vi "recouple_modes.vi"(10 "Decoupled":sgl[](array[numeric]) format="%#_3f") -> (2 "Output":sgl[](array[numeric]) format="%#_3g")   [LabVIEW 2013]
panel:
  # "Inverse of decouple_modes.vi"
  # "----------XY----------"
  # "----------RxRy----------"
  # "Z"
  # "Rz"
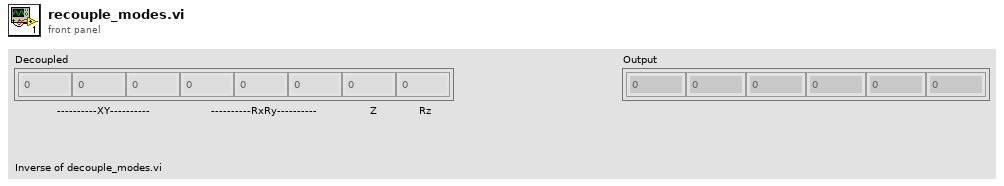
[diagram p1: front panel]
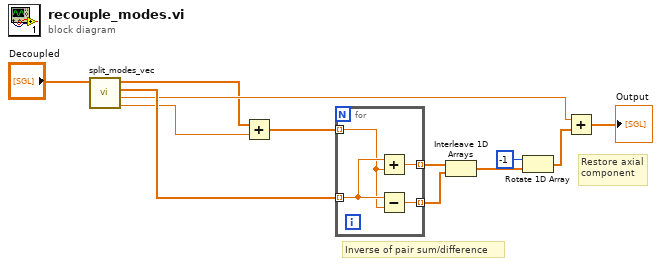
[diagram p0: block diagram]
diagram:
  # "Restore axial\ncomponent"
  # "Inverse of pair sum/difference"
  n1 = call "split_modes_vec.vi"("Decoupled"="Decoupled") -> ("Rz"=w1:sgl, "Z"=w3:sgl, "Rx Ry"=w4:sgl[], "XY"=w2:sgl[])  [unwired: 7 in]
  n2 = Add(x=w2, y=w1) -> (x+y=w7:sgl[])
  n3 = for {
    tunnel: w7 -> [w15] mode=indexing
    tunnel: w4 -> [w16] mode=indexing
    tunnel: [w14] -> w12 mode=indexing
    tunnel: [w13] -> w11 mode=indexing
    n4 = Add(x=w16, y=w15) -> (x+y=w14:sgl)
    n5 = Subtract(x=w16, y=w15) -> (x-y=w13:sgl)
  }
  n6 = Interleave 1D Arrays(w12, w11) -> (w9:sgl[])
  n7 = Rotate 1D Array(1:w9, 2:-1 ("n")) -> (0:w8:sgl[])
  n8 = Add(x=w3, y=w8) -> (x+y=→"Output":sgl[])
